vi "distance limit.vi"(0 "Encoder Rate":dbl, 1 "Encoder Distance":dbl, 2 "Desired Rate":dbl, 3 "Forward Limit":dbl, 5 "Reverse Limit":dbl) -> (4 "At Distance Limit":bool, 6 "Encoder Rate Out":dbl, 7 "Output Rate":dbl)   [LabVIEW 2014]
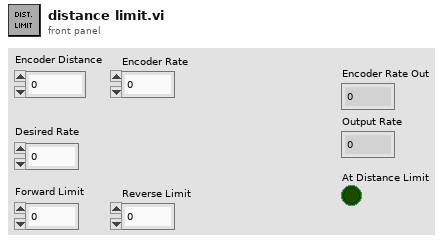
[diagram p1: front panel]
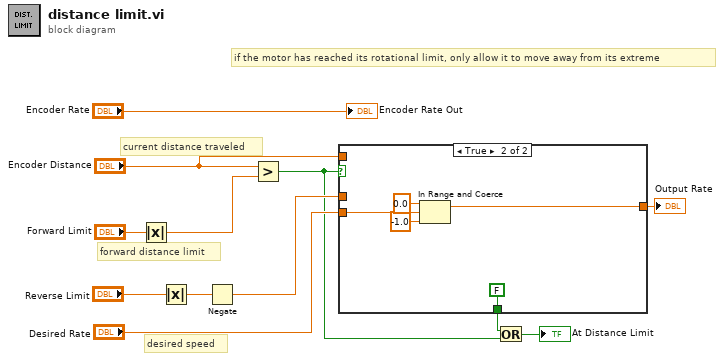
[diagram p0: block diagram]
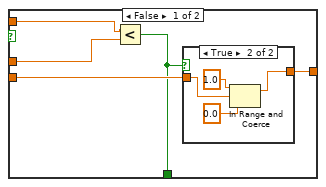
[diagram p2: hidden frame]
diagram:
  # "desired speed"
  # "forward distance limit"
  # "current distance traveled"
  # "if the motor has reached its rotational limit, only allow it to move away from its extreme"
  n1 = Absolute Value(x="Forward Limit") -> (abs(x)=w7:dbl)
  n2 = Absolute Value(x="Reverse Limit") -> (abs(x)=w5:dbl)
  n3 = Negate(x=w5) -> (-x=w4:dbl)
  n4 = Greater?(x="Encoder Distance", y=w7) -> (0:w2:bool)
  n5 = case shown="True" w2 {
    tunnel: "Desired Rate" -> [w16 w27]
    tunnel: "Encoder Distance" -> [w17 _]
    tunnel: [w15 w24] -> w8
    tunnel: w4 -> [w14 _]
    tunnel: [w13 FALSE] -> w3
    frame False {
      n6 = Less?(x=w17, y=w14) -> (x < y?=w13:bool)
      n7 = case shown="True" w13 {
        tunnel: w16 -> [w18 w20]
        tunnel: [w18 w19] -> w15
        frame False {
        }
        frame True {
          n8 = In Range and Coerce(upper limit=1.0, x=w20, lower limit=0.0) -> (coerced(x)=w19:dbl)  [unwired: 1 out]
        }
      }
    }
    frame True {
      n9 = In Range and Coerce(upper limit=0.0, x=w27, lower limit=-1.0) -> (coerced(x)=w24:dbl)  [unwired: 1 out]
    }
  }
  "Output Rate" <- w8
  n10 = Or(x=w3, y=w2) -> (x .or. y?=→"At Distance Limit":bool)
  "Encoder Rate Out" <- "Encoder Rate"
